vi "LaserWrite.vi"(7 "error in (no error)":errorcluster, 9 "Command":string="WX,PRG=0000,BLK=000,CharacterString=\"HelloWord\"", 10 "connection ID":refnum<k5>) -> (0 "error out":errorcluster, 1 "Sended":bool, 2 "Command out":string="WX,PRG=0000,BLK=000,CharacterString=\"HelloWord\"", 3 "connection ID out":refnum<k5>)   [LabVIEW 2018]
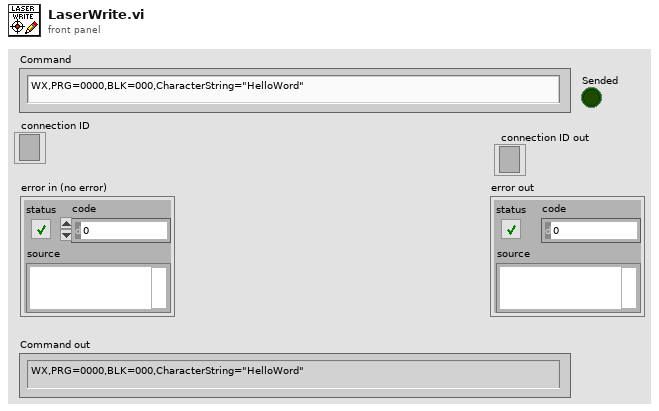
[diagram p1: front panel]
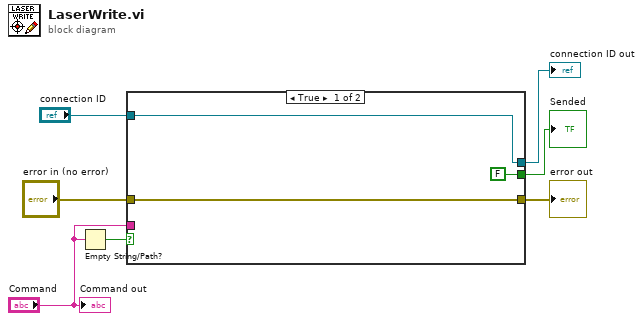
[diagram p0: block diagram]
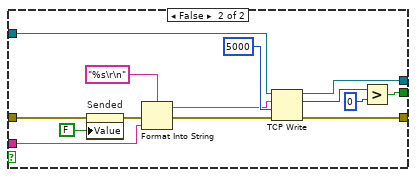
[diagram p2: hidden frame]
diagram:
  n1 = Empty String/Path?(string/path="Command") -> (empty?=w1:bool)
  n2 = case shown="True" w1 {
    tunnel: "Command" -> [_ w23]
    tunnel: "error in (no error)" -> [w9 w15]
    tunnel: [w9 w14] -> w6
    tunnel: [FALSE w13] -> w5
    tunnel: [w10 w12] -> w4
    tunnel: "connection ID" -> [w10 w11]
    frame True {
    }
    frame False {
      n3 = property on="Sended" class="Bool (strict)"(error in=w15, "Value"=FALSE ("Sended")) -> (error out=w17:errorcluster)  [unwired: 1 in, 1 out]
      n4 = Format Into String "Format Into String"(format string="%s\r\n", error in=w17, w23) -> (resulting string=w21:string, error out=w20:errorcluster)  [unwired: 1 in]
      n5 = TCP Write(connection ID=w11, data in=w21, error in (no error)=w20, 9:5000 ("timeout ms (25000)")) -> (connection ID out=w12:refnum<k5>, bytes written=w19:i32, error out=w14:errorcluster)
      n6 = Greater?(x=w19, y=0) -> (0:w13:bool)
    }
  }
  "error out" <- w6
  "Sended" <- w5
  "connection ID out" <- w4
  "Command out" <- "Command"
